vi "RSD.vi"(2 "C":bool, 3 "S":bool, 4 "D":bool, 5 "R":bool) -> (0 "!Q":bool, 1 "Q":bool)   [LabVIEW 2013]
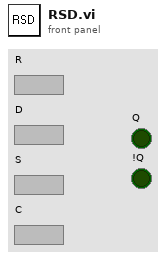
[diagram p1: front panel]
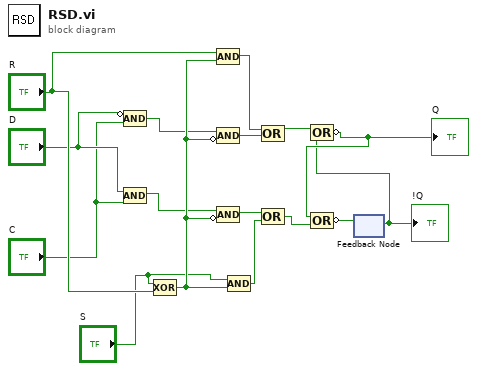
[diagram p0: block diagram]
diagram:
  n1 = Compound Arithmetic op=AND(invert "D", "C") -> (w13:bool)
  n2 = Compound Arithmetic op=AND("D", "C") -> (w12:bool)
  n3 = Compound Arithmetic op=XOR("S", "R") -> (w15:bool)
  n4 = Compound Arithmetic op=AND("R", w15) -> (w10:bool)
  n5 = Compound Arithmetic op=AND(w13, invert w15) -> (w11:bool)
  n6 = Compound Arithmetic op=AND(w12, invert w15) -> (w8:bool)
  n7 = Compound Arithmetic op=AND("S", w15) -> (w9:bool)
  n8 = Compound Arithmetic op=OR(w10, w11) -> (w6:bool)
  n9 = Compound Arithmetic op=OR(w8, w9) -> (w7:bool)
  n10 = feedback #1() -> (w3:bool)  [unwired: 1 in]
  "!Q" <- w3
  n11 = Compound Arithmetic op=OR(w6, w3) -> (invert w5:bool)
  "Q" <- w5
  n12 = Compound Arithmetic op=OR(w5, w7) -> (invert w4:bool)
  n13 = feedback-in #1(w4) -> ()
